vi "main-for-loop-V2.vi"() -> ()   [LabVIEW 2024]
uses:
  controls/thermocouple-input-cluster.ctl
  controls/analog-input-cluster.ctl
  controls/analog-output-cluster.ctl
  controls/digitial-input-cluster.ctl
  controls/digital-output-cluster.ctl
  controls/adam-module-select-tab.ctl
  controls/adam-5000-serial-settings.ctl
  controls/adam-5000-cmd-response.ctl
  controls/state-enum.ctl
  controls/adam-5000-all-chassis-data.ctl
  controls/adam-5000-all-module-datas.ctl
  controls/adam-5000-chassis-cmd-ack.ctl
  <vilib>/Instr/_visa.llb/VISA Configure Serial Port (Instr).vi
  <vilib>/Instr/_visa.llb/VISA Flush IO Buffer Mask.ctl
  controls/adam-5000-module-cmd-ack.ctl
panel:
  out "cmd-response:7":T1
  out "status-indicator:7":cluster{"Sampling":bool, "Ack":bool}
  in  "Slot 7: Module Type":T2(ring)=enum."empty"
  out "slot: 7":T3
  in  "7:Digital Outputs":T4
  out "7:Digital Inputs":T5
  in  "7:Analog Outputs":T6
  out "7:Analog Inputs":T7
  out "7:Thermocouple Inputs (degC)":T8
  out "cmd-response:6":T1
  out "status-indicator:6":cluster{"Sampling":bool, "Ack":bool}
  in  "Slot 6: Module Type":T2(ring)=enum."empty"
  out "slot: 6":T3
  in  "6:Digital Outputs":T4
  out "6:Digital Inputs":T5
  in  "6:Analog Outputs":T6
  out "6:Analog Inputs":T7
  out "6:Thermocouple Inputs (degC)":T8
  out "cmd-response:5":T1
  out "status-indicator:5":cluster{"Sampling":bool, "Ack":bool}
  in  "Slot 5: Module Type":T2(ring)=enum."Analog Output"
  out "slot: 5":T3
  in  "5:Digital Outputs":T4
  out "5:Digital Inputs":T5
  in  "5:Analog Outputs":T6
  out "5:Analog Inputs":T7
  out "5:Thermocouple Inputs (degC)":T8
  out "cmd-response:4":T1
  out "status-indicator:4":cluster{"Sampling":bool, "Ack":bool}
  in  "Slot 4: Module Type":T2(ring)=enum."Power Relay"
  out "slot: 4":T3
  in  "4:Digital Outputs":T4
  out "4:Digital Inputs":T5
  in  "4:Analog Outputs":T6
  out "4:Analog Inputs":T7
  out "4:Thermocouple Inputs (degC)":T8
  out "cmd-response:3":T1
  out "status-indicator:3":cluster{"Sampling":bool, "Ack":bool}
  in  "Slot 3: Module Type":T2(ring)=enum."Thermocouple"
  out "slot: 3":T3
  in  "3:Digital Outputs":T4
  out "3:Digital Inputs":T5
  in  "3:Analog Outputs":T6
  out "3:Analog Inputs":T7
  out "3:Thermocouple Inputs (degC)":T8
  out "cmd-response:2":T1
  out "status-indicator:2":cluster{"Sampling":bool, "Ack":bool}
  in  "Slot 2: Module Type":T2(ring)=enum."Analog Input"
  out "slot: 2":T3
  in  "2:Digital Outputs":T4
  out "2:Digital Inputs":T5
  in  "2:Analog Outputs":T6
  out "2:Analog Inputs":T7
  out "2:Thermocouple Inputs (degC)":T8
  out "cmd-response:1":T1
  out "status-indicator:1":cluster{"Sampling":bool, "Ack":bool}
  in  "Slot 1: Module Type":T2(ring)=enum."Thermocouple"
  out "slot: 1":T3
  in  "1:Digital Outputs":T4
  out "1:Digital Inputs":T5
  in  "1:Analog Outputs":T6
  out "1:Analog Inputs":T7
  out "1:Thermocouple Inputs (degC)":T8
  out "cmd-response:0":T1
  out "status-indicator:0":cluster{"Sampling":bool, "Ack":bool}
  in  "Slot 0: Module Type":T2(ring)=enum."Analog Input"
  out "slot: 0":T3
  in  "0:Digital Outputs":T4
  out "0:Digital Inputs":T5
  in  "0:Analog Outputs:":T6
  out "0:Analog Inputs":T7
  out "0:Thermocouple Inputs (degC)":T8
  out "Current Slot":i32
  in  "Chassis Settings":T9={"VISA resource name"="COM10", "baud rate (19200)"=19200, "Chassis ID"=1}
  in  "Debug Mode":bool
  out "Loop Time (mS)":u32
  out "Loop Counter":i32
  out "Write Success":bool
  out "error IO":errorcluster
  out "error":errorcluster
  in  "exit":bool
  # "ADAM 5000 Controller"
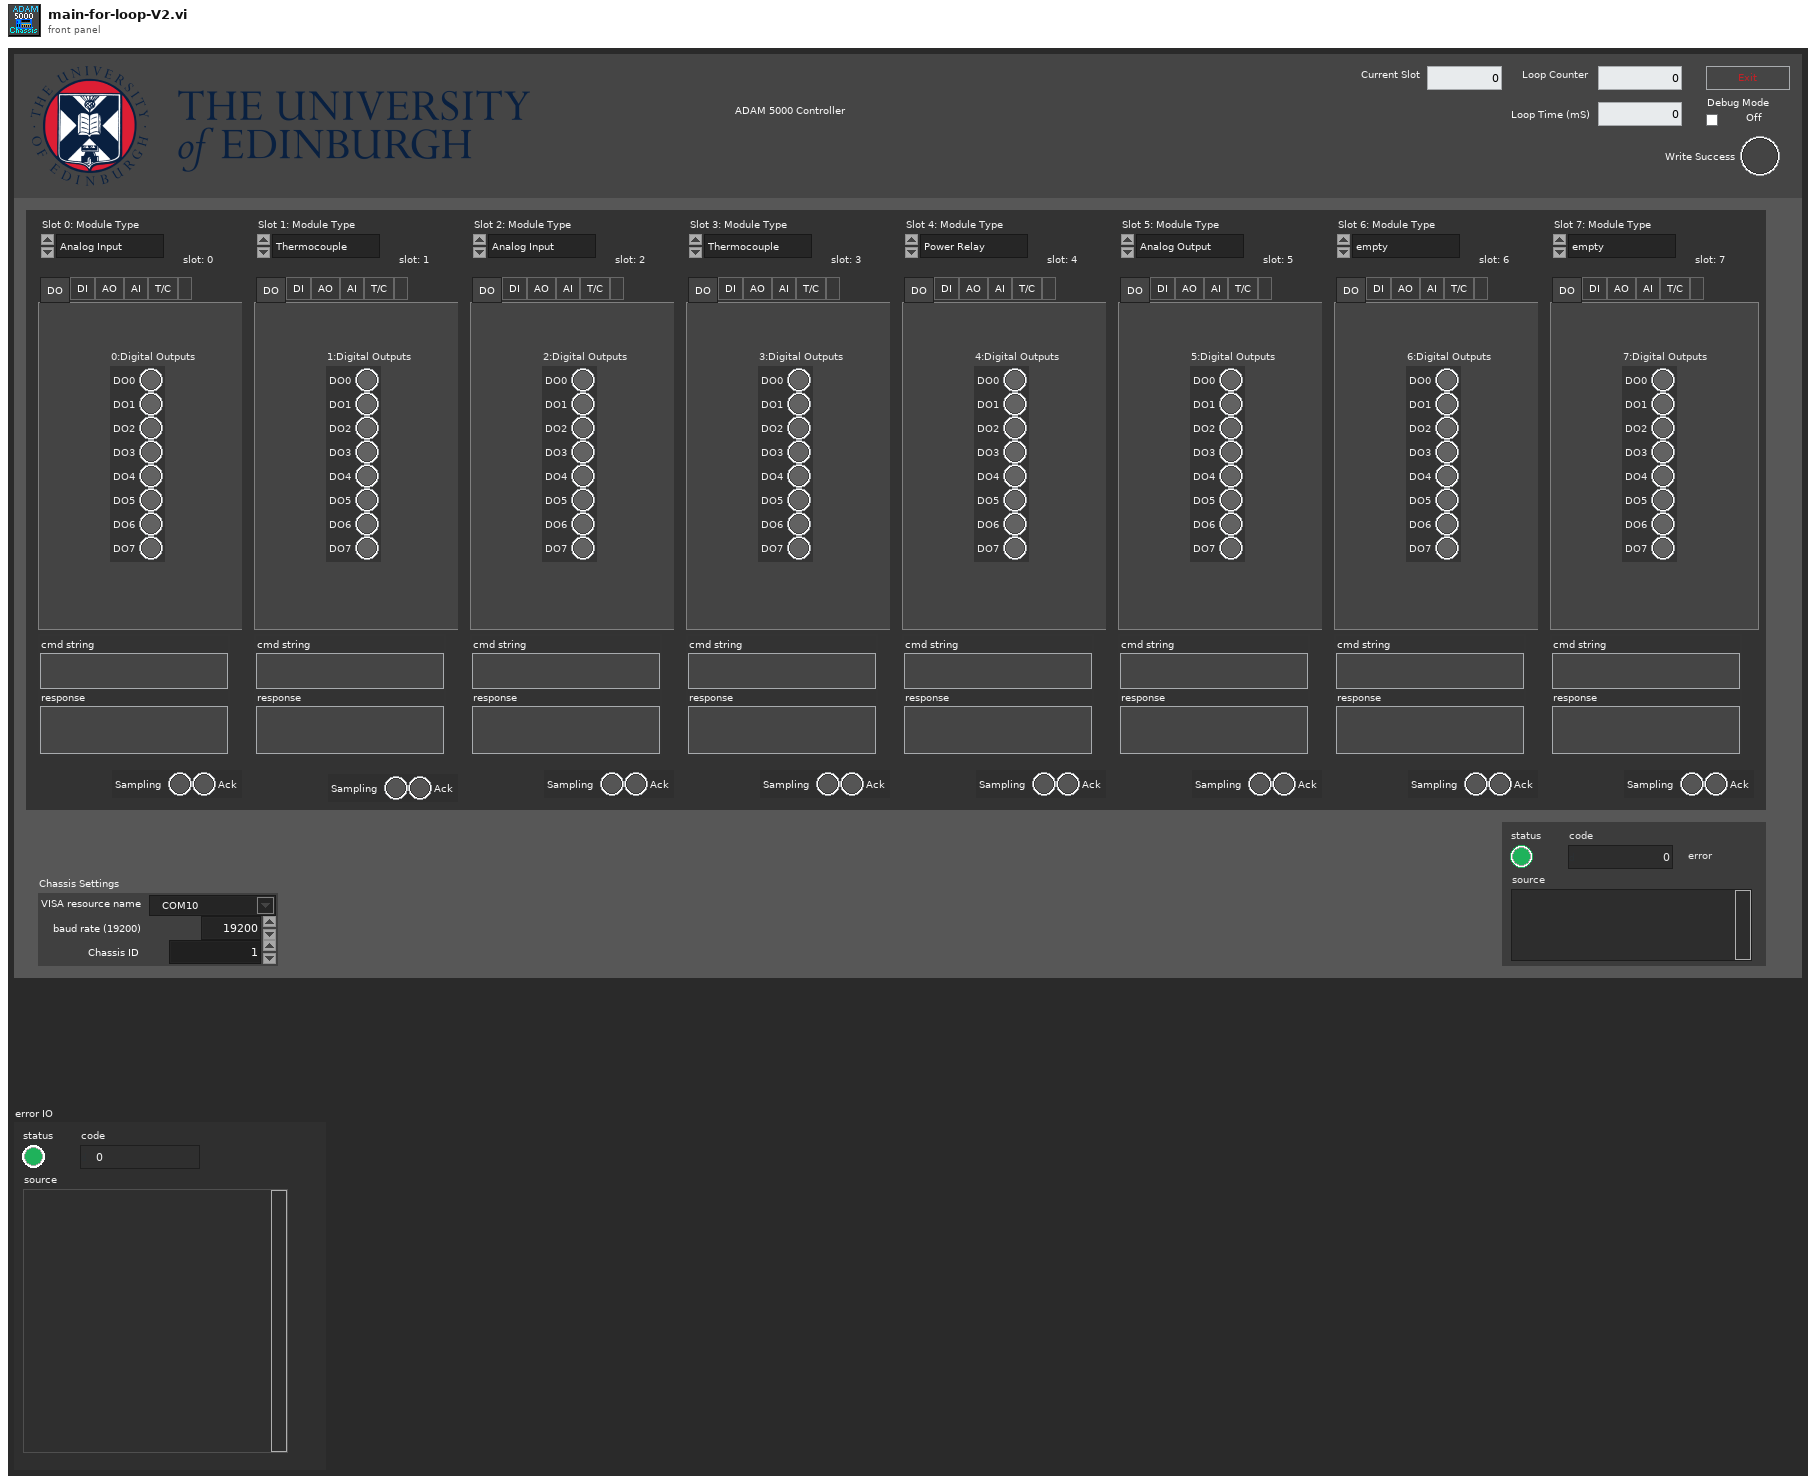
[diagram p1: front panel]
types:
  T1 = typedef "adam-5000-cmd-response.ctl" = cluster{"cmd string":string, "response":string}
  T2 = enum16{"Digital Output", "Digital Input", "Analog Output", "Analog Input", "Thermocouple", "Power Relay", "empty"}
  T3 = typedef "adam-module-select-tab.ctl" = enum32{"DO", "DI", "AO", "AI", "T/C", ""}
  T4 = typedef "digital-output-cluster.ctl" = cluster{"DO0":bool, "DO1":bool, "DO2":bool, "DO3":bool, "DO4":bool, "DO5":bool, "DO6":bool, "DO7":bool}
  T5 = typedef "digitial-input-cluster.ctl" = cluster{"DI0":bool, "DI1":bool, "DI2":bool, "DI3":bool, "DI4":bool, "DI5":bool, "DI6":bool, "DI7":bool}
  T6 = typedef "analog-output-cluster.ctl" = cluster{"AO0":dbl, "AO1":dbl, "AO2":dbl, "AO3":dbl}
  T7 = typedef "analog-input-cluster.ctl" = cluster{"AI0":dbl, "AI1":dbl, "AI2":dbl, "AI3":dbl, "AI4":dbl, "AI5":dbl, "AI6":dbl, "AI7":dbl}
  T8 = typedef "thermocouple-input-cluster.ctl" = cluster{"TC0":dbl, "TC1":dbl, "TC2":dbl, "TC3":dbl, "TC4":dbl, "TC5":dbl, "TC6":dbl}
  T9 = typedef "adam-5000-serial-settings.ctl" = cluster{"VISA resource name":refnum<visa-resource-name>, "baud rate (19200)":u32, "Chassis ID":u8}
  T10 = typedef "adam-5000-chassis-cmd-ack.ctl" = cluster{"cmd-response:0":T1, "cmd-response:1":T1, "cmd-response:2":T1, "cmd-response:3":T1, "cmd-response:4":T1, "cmd-response:5":T1, "cmd-response:6":T1, "cmd-response:7":T1}
  T11 = typedef "adam-5000-all-chassis-data.ctl" = cluster{"slot:0":T12, "slot:1":T12, "slot:2":T12, "slot:3":T12, "slot:4":T12, "slot:5":T12, "slot:6":T12, "slot:7":T12}
  T12 = typedef "adam-5000-all-module-datas.ctl" = cluster{"Digital Outputs":T4, "Digital Inputs":T5, "Analog Outputs":T6, "Analog Inputs":T7, "Thermocouple Inputs (degC)":T8}
  T13 = typedef "state-enum.ctl" = enum16{"init", "manual", "start", "run", "hold", "stop", ""}
  T14 = cluster{"0:Digital Outputs":T4, "1:Digital Outputs":T4, "2:Digital Outputs":T4, "3:Digital Outputs":T4, "4:Digital Outputs":T4, "5:Digital Outputs":T4, "6:Digital Outputs":T4, "7:Digital Outputs":T4}
  T15 = cluster{"Slot 0: Module Type":enum16{"Digital Output", "Digital Input", "Analog Output", "Analog Input", "Thermocouple", "Power Relay", "empty"}, "Slot 1: Module Type":enum16{"Digital Output", "Digital Input", "Analog Output", "Analog Input", "Thermocouple", "Power Relay", "empty"}, "Slot 2: Module Type":enum16{"Digital Output", "Digital Input", "Analog Output", "Analog Input", "Thermocouple", "Power Relay", "empty"}, "Slot 3: Module Type":enum16{"Digital Output", "Digital Input", "Analog Output", "Analog Input", "Thermocouple", "Power Relay", "empty"}, "Slot 4: Module Type":enum16{"Digital Output", "Digital Input", "Analog Output", "Analog Input", "Thermocouple", "Power Relay", "empty"}, "Slot 5: Module Type":enum16{"Digital Output", "Digital Input", "Analog Output", "Analog Input", "Thermocouple", "Power Relay", "empty"}, "Slot 6: Module Type":enum16{"Digital Output", "Digital Input", "Analog Output", "Analog Input", "Thermocouple", "Power Relay", "empty"}, "Slot 7: Module Type":enum16{"Digital Output", "Digital Input", "Analog Output", "Analog Input", "Thermocouple", "Power Relay", "empty"}}
  T16 = cluster{"status-indicator:0":refnum<vi>, "status-indicator:1":refnum<vi>, "status-indicator:2":refnum<vi>, "status-indicator:3":refnum<vi>, "status-indicator:4":refnum<vi>, "status-indicator:5":refnum<vi>, "status-indicator:6":refnum<vi>, "status-indicator:7":refnum<vi>}
  T17 = cluster{"0:Analog Outputs:":T6, "1:Analog Outputs":T6, "2:Analog Outputs":T6, "3:Analog Outputs":T6, "4:Analog Outputs":T6, "5:Analog Outputs":T6, "6:Analog Outputs":T6, "7:Analog Outputs":T6}
  T18 = enum16{"Digital Output", "Digital Input", "Analog Output", "Analog Input", "Thermocouple", "Power Relay", "empty"}[]
  T19 = cluster{"[0]":T3, "[1]":T3, "[2]":T3, "[3]":T3, "[4]":T3, "[5]":T3, "[6]":T3, "[7]":T3, "[8]":T3}
  T20 = cluster{"[0]":T1, "[1]":T1, "[2]":T1, "[3]":T1, "[4]":T1, "[5]":T1, "[6]":T1, "[7]":T1, "[8]":T1}
  T21 = cluster{"[0]":T12, "[1]":T12, "[2]":T12, "[3]":T12, "[4]":T12, "[5]":T12, "[6]":T12, "[7]":T12, "[8]":T12}
  T22 = typedef "adam-5000-module-cmd-ack.ctl" = cluster{"cmd out":string, "acknowledge char":string}
  T23 = cluster{"[0]":T22, "[1]":T22, "[2]":T22, "[3]":T22, "[4]":T22, "[5]":T22, "[6]":T22, "[7]":T22, "[8]":T22}
  T24 = typedef "VISA Flush IO Buffer Mask.ctl" = u16
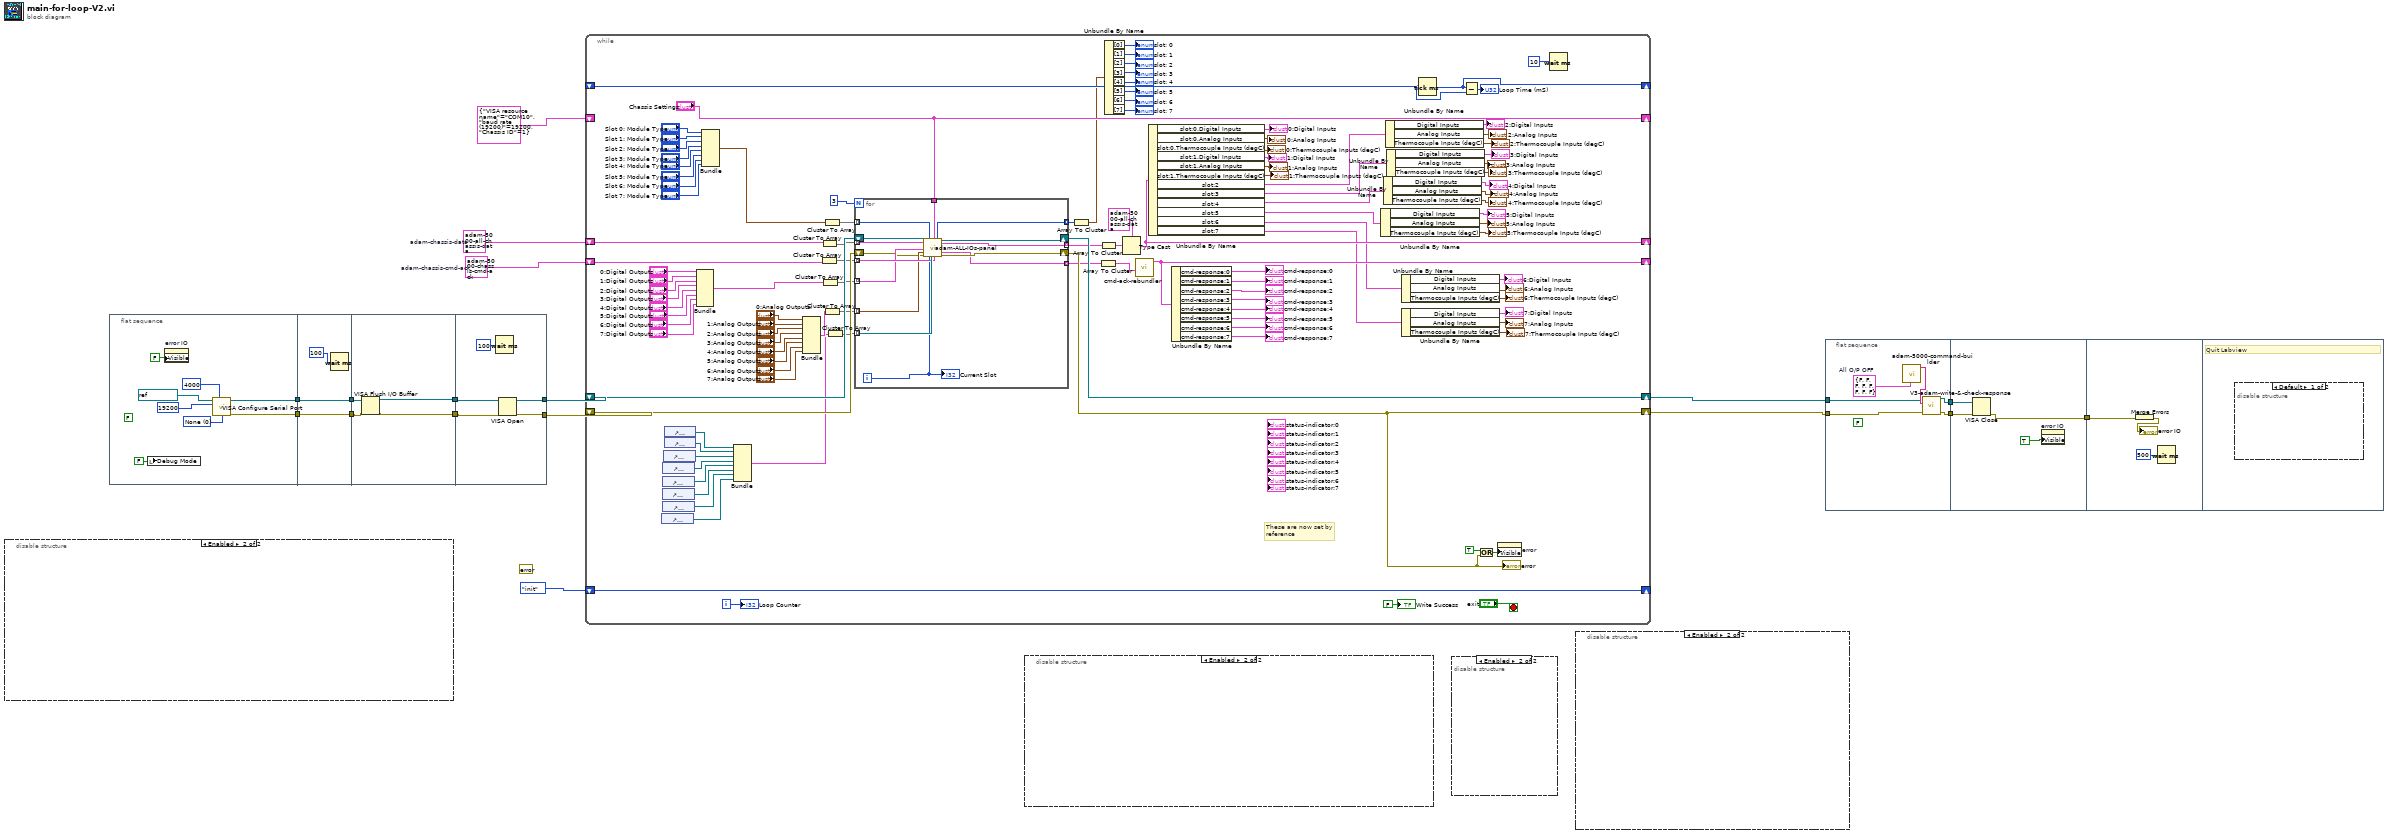
[diagram p0: block diagram]
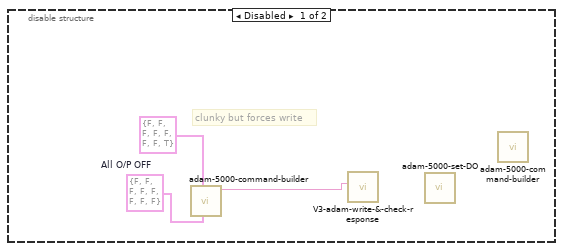
[diagram p2: hidden frame]
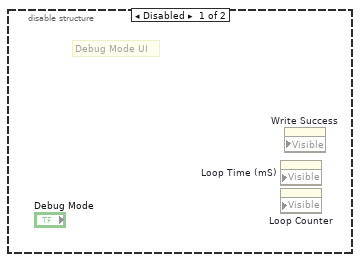
[diagram p3: hidden frame]
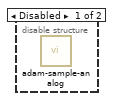
[diagram p4: hidden frame]
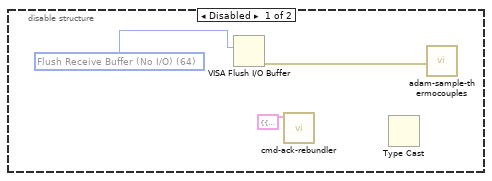
[diagram p5: hidden frame]
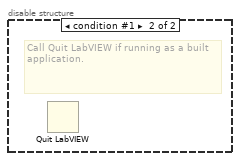
[diagram p6: hidden frame]
diagram:
  w1 = T10 {"cmd-response:0"={"cmd string"="", "response"=""}, "cmd-response:1"={"cmd string"="", "response"=""}, "cmd-response:2"={"cmd string"="", "response"=""}, "cmd-response:3"={"cmd string"="", "response"=""}, "cmd-response:4"={"cmd string"="", "response"=""}, "cmd-response:5"={"cmd string"="", "response"=""}, "cmd-response:6"={"cmd string"="", "response"=""}, "cmd-response:7"={"cmd string"="", "response"=""}}  # adam-chassis-cmd-ack
  w2 = T11 {"slot:0"={"Digital Outputs"={"DO0"=FALSE, "DO1"=FALSE, "DO2"=FALSE, "DO3"=FALSE, "DO4"=FALSE, "DO5"=FALSE, "DO6"=FALSE, "DO7"=FALSE}, "Digital Inputs"={"DI0"=FALSE, "DI1"=FALSE, "DI2"=FALSE, "DI3"=FALSE, "DI4"=FALSE, "DI5"=FALSE, "DI6"=FALSE, "DI7"=FALSE}, "Analog Outputs"={"AO0"=0.0, "AO1"=0.0, "AO2"=0.0, "AO3"=0.0}, "Analog Inputs"={"AI0"=0.0, "AI1"=0.0, "AI2"=0.0, "AI3"=0.0, "AI4"=0.0, "AI5"=0.0, "AI6"=0.0, "AI7"=0.0}, "Thermocouple Inputs (degC)"={"TC0"=0.0, "TC1"=0.0, "TC2"=0.0, "TC3"=0.0, "TC4"=0.0, "TC5"=0.0, "TC6"=0.0}}, "slot:1"={"Digital Outputs"={"DO0"=FALSE, "DO1"=FALSE, "DO2"=FALSE, "DO3"=FALSE, "DO4"=FALSE, "DO5"=FALSE, "DO6"=FALSE, "DO7"=FALSE}, "Digital Inputs"={"DI0"=FALSE, "DI1"=FALSE, "DI2"=FALSE, "DI3"=FALSE, "DI4"=FALSE, "DI5"=FALSE, "DI6"=FALSE, "DI7"=FALSE}, "Analog Outputs"={"AO0"=0.0, "AO1"=0.0, "AO2"=0.0, "AO3"=0.0}, "Analog Inputs"={"AI0"=0.0, "AI1"=0.0, "AI2"=0.0, "AI3"=0.0, "AI4"=0.0, "AI5"=0.0, "AI6"=0.0, "AI7"=0.0}, "Thermocouple Inputs (degC)"={"TC0"=0.0, "TC1"=0.0, "TC2"=0.0, "TC3"=0.0, "TC4"=0.0, "TC5"=0.0, "TC6"=0.0}}, "slot:2"={"Digital Outputs"={"DO0"=FALSE, "DO1"=FALSE, "DO2"=FALSE, "DO3"=FALSE, "DO4"=FALSE, "DO5"=FALSE, "DO6"=FALSE, "DO7"=FALSE}, "Digital Inputs"={"DI0"=FALSE, "DI1"=FALSE, "DI2"=FALSE, "DI3"=FALSE, "DI4"=FALSE, "DI5"=FALSE, "DI6"=FALSE, "DI7"=FALSE}, "Analog Outputs"={"AO0"=0.0, "AO1"=0.0, "AO2"=0.0, "AO3"=0.0}, "Analog Inputs"={"AI0"=0.0, "AI1"=0.0, "AI2"=0.0, "AI3"=0.0, "AI4"=0.0, "AI5"=0.0, "AI6"=0.0, "AI7"=0.0}, "Thermocouple Inputs (degC)"={"TC0"=0.0, "TC1"=0.0, "TC2"=0.0, "TC3"=0.0, "TC4"=0.0, "TC5"=0.0, "TC6"=0.0}}, "slot:3"={"Digital Outputs"={"DO0"=FALSE, "DO1"=FALSE, "DO2"=FALSE, "DO3"=FALSE, "DO4"=FALSE, "DO5"=FALSE, "DO6"=FALSE, "DO7"=FALSE}, "Digital Inputs"={"DI0"=FALSE, "DI1"=FALSE, "DI2"=FALSE, "DI3"=FALSE, "DI4"=FALSE, "DI5"=FALSE, "DI6"=FALSE, "DI7"=FALSE}, "Analog Outputs"={"AO0"=0.0, "AO1"=0.0, "AO2"=0.0, "AO3"=0.0}, "Analog Inputs"={"AI0"=0.0, "AI1"=0.0, "AI2"=0.0, "AI3"=0.0, "AI4"=0.0, "AI5"=0.0, "AI6"=0.0, "AI7"=0.0}, "Thermocouple Inputs (degC)"={"TC0"=0.0, "TC1"=0.0, "TC2"=0.0, "TC3"=0.0, "TC4"=0.0, "TC5"=0.0, "TC6"=0.0}}, "slot:4"={"Digital Outputs"={"DO0"=FALSE, "DO1"=FALSE, "DO2"=FALSE, "DO3"=FALSE, "DO4"=FALSE, "DO5"=FALSE, "DO6"=FALSE, "DO7"=FALSE}, "Digital Inputs"={"DI0"=FALSE, "DI1"=FALSE, "DI2"=FALSE, "DI3"=FALSE, "DI4"=FALSE, "DI5"=FALSE, "DI6"=FALSE, "DI7"=FALSE}, "Analog Outputs"={"AO0"=0.0, "AO1"=0.0, "AO2"=0.0, "AO3"=0.0}, "Analog Inputs"={"AI0"=0.0, "AI1"=0.0, "AI2"=0.0, "AI3"=0.0, "AI4"=0.0, "AI5"=0.0, "AI6"=0.0, "AI7"=0.0}, "Thermocouple Inputs (degC)"={"TC0"=0.0, "TC1"=0.0, "TC2"=0.0, "TC3"=0.0, "TC4"=0.0, "TC5"=0.0, "TC6"=0.0}}, "slot:5"={"Digital Outputs"={"DO0"=FALSE, "DO1"=FALSE, "DO2"=FALSE, "DO3"=FALSE, "DO4"=FALSE, "DO5"=FALSE, "DO6"=FALSE, "DO7"=FALSE}, "Digital Inputs"={"DI0"=FALSE, "DI1"=FALSE, "DI2"=FALSE, "DI3"=FALSE, "DI4"=FALSE, "DI5"=FALSE, "DI6"=FALSE, "DI7"=FALSE}, "Analog Outputs"={"AO0"=0.0, "AO1"=0.0, "AO2"=0.0, "AO3"=0.0}, "Analog Inputs"={"AI0"=0.0, "AI1"=0.0, "AI2"=0.0, "AI3"=0.0, "AI4"=0.0, "AI5"=0.0, "AI6"=0.0, "AI7"=0.0}, "Thermocouple Inputs (degC)"={"TC0"=0.0, "TC1"=0.0, "TC2"=0.0, "TC3"=0.0, "TC4"=0.0, "TC5"=0.0, "TC6"=0.0}}, "slot:6"={"Digital Outputs"={"DO0"=FALSE, "DO1"=FALSE, "DO2"=FALSE, "DO3"=FALSE, "DO4"=FALSE, "DO5"=FALSE, "DO6"=FALSE, "DO7"=FALSE}, "Digital Inputs"={"DI0"=FALSE, "DI1"=FALSE, "DI2"=FALSE, "DI3"=FALSE, "DI4"=FALSE, "DI5"=FALSE, "DI6"=FALSE, "DI7"=FALSE}, "Analog Outputs"={"AO0"=0.0, "AO1"=0.0, "AO2"=0.0, "AO3"=0.0}, "Analog Inputs"={"AI0"=0.0, "AI1"=0.0, "AI2"=0.0, "AI3"=0.0, "AI4"=0.0, "AI5"=0.0, "AI6"=0.0, "AI7"=0.0}, "Thermocouple Inputs (degC)"={"TC0"=0.0, "TC1"=0.0, "TC2"=0.0, "TC3"=0.0, "TC4"=0.0, "TC5"=0.0, "TC6"=0.0}}, "slot:7"={"Digital Outputs"={"DO0"=FALSE, "DO1"=FALSE, "DO2"=FALSE, "DO3"=FALSE, "DO4"=FALSE, "DO5"=FALSE, "DO6"=FALSE, "DO7"=FALSE}, "Digital Inputs"={"DI0"=FALSE, "DI1"=FALSE, "DI2"=FALSE, "DI3"=FALSE, "DI4"=FALSE, "DI5"=FALSE, "DI6"=FALSE, "DI7"=FALSE}, "Analog Outputs"={"AO0"=0.0, "AO1"=0.0, "AO2"=0.0, "AO3"=0.0}, "Analog Inputs"={"AI0"=0.0, "AI1"=0.0, "AI2"=0.0, "AI3"=0.0, "AI4"=0.0, "AI5"=0.0, "AI6"=0.0, "AI7"=0.0}, "Thermocouple Inputs (degC)"={"TC0"=0.0, "TC1"=0.0, "TC2"=0.0, "TC3"=0.0, "TC4"=0.0, "TC5"=0.0, "TC6"=0.0}}}  # adam-chassis-data
  (unwired) errorcluster {"status"=FALSE, "code"=0, "source"=""} ("error")
  n1 = disable-structure shown="Enabled" {
    frame Disabled {
      w20 = T4 {"DO0"=FALSE, "DO1"=FALSE, "DO2"=FALSE, "DO3"=FALSE, "DO4"=FALSE, "DO5"=FALSE, "DO6"=FALSE, "DO7"=FALSE}  # All O/P OFF
      # "clunky but forces write"
      n2 = call "adam-5000-command-builder.vi"("Output Control"=w20, "Current Output State"=T4 {"DO0"=FALSE, "DO1"=FALSE, "DO2"=FALSE, "DO3"=FALSE, "DO4"=FALSE, "DO5"=FALSE, "DO6"=FALSE, "DO7"=TRUE}) -> ("Command Out"=w19:string)  [unwired: 7 in, 2 out]
      n3 = call "V3-adam-write-&-check-response.vi"("write buffer"=w19) -> ("VISA resource name"=w18:refnum<visa-resource-name>)  [unwired: 5 in, 5 out]
      n4 = call "adam-5000-set-DO.vi"() -> ()  [unwired: 6 in, 6 out]
      n5 = call "adam-5000-command-builder.vi"() -> ()  [unwired: 9 in, 3 out]
    }
    frame Enabled {
    }
  }
  n6 = flat-sequence {
    tunnel: [w28] -> w11
    tunnel: [w27] -> w10
    tunnel: w11 -> [w32]
    tunnel: [w32] -> w9
    tunnel: w10 -> [w31]
    tunnel: [w31] -> w8
    tunnel: w9 -> [w36]
    tunnel: [w34] -> w7
    tunnel: w8 -> [w35]
    tunnel: [w33] -> w6
    tunnel: w7 -> [w40]
    tunnel: w6 -> [w39]
    tunnel: [w38] -> w5
    tunnel: [w37] -> w4
    frame #0 {
      w25 = u16 0 items=["None", "XON/XOFF", "RTS/CTS", "XON/XOFF & RTS/CTS", "DTR/DSR", "XON/XOFF & DTR/DSR"] ("flow control (0:none)")
      (unwired) FALSE ("V1")
      n7 = local write "Debug Mode"(FALSE ("Debug Mode")) -> ()
      n8 = property on="error IO" class="Clust (strict)"("Visible"=FALSE) -> ()  [unwired: 2 in, 2 out]
      n9 = call-poly "VISA Configure Serial Port"("VISA resource name"=refnum<visa-resource-name> "COM10", "timeout (10sec)"=u32 4000, "baud rate (9600)"=u32 19200, "flow control (0:none)"=w25) -> ("VISA resource name out"=w28:refnum<visa-resource-name>, "error out"=w27:errorcluster)  [unwired: 10 in]
    }
    frame #1 {
      n10 = Wait (ms)(milliseconds to wait=u32 100) -> ()  [unwired: 1 out]
    }
    frame #2 {
      n11 = VISA Flush I/O Buffer(VISA resource name=w36, error in (no error)=w35) -> (VISA resource name out=w34:refnum<visa-resource-name>, error out=w33:errorcluster)  [unwired: 1 in]
    }
    frame #3 {
      n12 = Wait (ms)(milliseconds to wait=u32 100) -> ()  [unwired: 1 out]
      n13 = VISA Open(error in (no error)=w39, VISA resource name=w40) -> (VISA resource name=w38:refnum<visa-resource-name>, error out=w37:errorcluster)  [unwired: 3 in]
    }
  }
  n14 = while {
    shift-right: [w148] -> _
    shift-left: state-enum."init" ("state-enum") -> [w148]
    shift-right: [w116] -> w16
    shift-left: w4 -> [w130]
    shift-right: [w151] -> _
    shift-left: _ -> [w153]
    shift-right: ["Chassis Settings"] -> _
    shift-left: T9 {"VISA resource name"="COM10", "baud rate (19200)"=19200, "Chassis ID"=1} ("Chassis Settings") -> [_]
    shift-right: [w129] -> w3
    shift-left: w5 -> [w131]
    shift-right: [w117] -> _
    shift-left: w2 -> [w128]
    shift-right: [w99] -> _
    shift-left: w1 -> [w126]
    i -> [w154]
    stop <- "exit" stop-if-true
    # "These are now set by\nreference"
    n15 = control-ref of="status-indicator:7"() -> (w42:refnum<vi>)
    n16 = control-ref of="status-indicator:4"() -> (w45:refnum<vi>)
    n17 = control-ref of="status-indicator:5"() -> (w44:refnum<vi>)
    n18 = control-ref of="status-indicator:3"() -> (w46:refnum<vi>)
    n19 = control-ref of="status-indicator:6"() -> (w43:refnum<vi>)
    n20 = control-ref of="status-indicator:2"() -> (w91:refnum<vi>)
    n21 = control-ref of="status-indicator:0"() -> (w112:refnum<vi>)
    n22 = control-ref of="status-indicator:1"() -> (w111:refnum<vi>)
    n23 = Bundle("0:Digital Outputs"="0:Digital Outputs", "1:Digital Outputs"="1:Digital Outputs", "2:Digital Outputs"="2:Digital Outputs", "3:Digital Outputs"="3:Digital Outputs", "4:Digital Outputs"="4:Digital Outputs", "5:Digital Outputs"="5:Digital Outputs", "6:Digital Outputs"="6:Digital Outputs", "7:Digital Outputs"="7:Digital Outputs") -> (w123:T14)  [unwired: 1 in]
    n24 = Bundle("Slot 0: Module Type"="Slot 0: Module Type", "Slot 1: Module Type"="Slot 1: Module Type", "Slot 2: Module Type"="Slot 2: Module Type", "Slot 3: Module Type"="Slot 3: Module Type", "Slot 4: Module Type"="Slot 4: Module Type", "Slot 5: Module Type"="Slot 5: Module Type", "Slot 6: Module Type"="Slot 6: Module Type", "Slot 7: Module Type"="Slot 7: Module Type") -> (w115:T15)  [unwired: 1 in]
    n25 = Bundle("status-indicator:0"=w112, "status-indicator:1"=w111, "status-indicator:2"=w91, "status-indicator:3"=w46, "status-indicator:4"=w45, "status-indicator:5"=w44, "status-indicator:6"=w43, "status-indicator:7"=w42) -> (w110:T16)  [unwired: 1 in]
    n26 = Bundle("0:Analog Outputs:"="0:Analog Outputs:", "1:Analog Outputs"="1:Analog Outputs", "2:Analog Outputs"="2:Analog Outputs", "3:Analog Outputs"="3:Analog Outputs", "4:Analog Outputs"="4:Analog Outputs", "5:Analog Outputs"="5:Analog Outputs", "6:Analog Outputs"="6:Analog Outputs", "7:Analog Outputs"="7:Analog Outputs") -> (w122:T17)  [unwired: 1 in]
    n27 = Cluster To Array(cluster=w126) -> (array=w125:T1[])
    n28 = Cluster To Array(cluster=w128) -> (array=w127:T12[])
    n29 = Cluster To Array(cluster=w123) -> (array=w124:T4[])
    n30 = Cluster To Array(cluster=w115) -> (array=w114:T18)
    n31 = Cluster To Array(cluster=w122) -> (array=w121:T6[])
    n32 = Cluster To Array(cluster=w110) -> (array=w109:refnum<vi>[])
    n33 = for {
      N: 3 -> [_]
      shift-right: [w160] -> w116
      shift-left: w130 -> [w161]
      shift-right: [w167] -> w129
      shift-left: w131 -> [w166]
      tunnel: w127 -> [w165] mode=indexing
      tunnel: w125 -> [w164] mode=indexing
      tunnel: w124 -> [w163] mode=indexing
      tunnel: w121 -> [w162] mode=indexing
      tunnel: "Chassis Settings" -> [w169]
      tunnel: w114 -> [w170] mode=indexing
      tunnel: w109 -> [w171] mode=indexing
      tunnel: [w168] -> w108 mode=indexing
      tunnel: [w159] -> w107 mode=indexing
      tunnel: [w158] -> w106 mode=indexing
      i -> [w157]
      n34 = call "adam-ALL-IOs-panel.vi"("VISA Refnum in"=w166, "ADAM-5000-data-current"=w165, "Digital Outputs"=w163, "Analog Outputs"=w162, "error in (no error)"=w161, "Module Type"=w170, "chassis-slot"=w157, "reference"=w171, "Chassis Settings"=w169, "cmd-response in"=w164) -> ("slot: x"=w168:T3, "VISA Refnum out"=w167:refnum<visa-resource-name>, "ADAM-5000-data-new"=w159:T12, "cmd-response out"=w158:T1, "error out"=w160:errorcluster)  [unwired: 5 in]
      "Current Slot" <- w157
    }
    "error" <- w116
    n35 = Array To Cluster(array=w108) -> (cluster=w113:T19)
    n36 = Array To Cluster(array=w106) -> (cluster=w98:T20)
    n37 = Array To Cluster(array=w107) -> (cluster=w119:T21)
    n38 = Unbundle By Name(w113) -> ("[0]"=→"slot: 0":T3, "[1]"=→"slot: 1":T3, "[2]"=→"slot: 2":T3, "[3]"=→"slot: 3":T3, "[4]"=→"slot: 4":T3, "[5]"=→"slot: 5":T3, "[6]"=→"slot: 6":T3, "[7]"=→"slot: 7":T3)
    n39 = Type Cast(type=T11 {"slot:0"={"Digital Outputs"={"DO0"=FALSE, "DO1"=FALSE, "DO2"=FALSE, "DO3"=FALSE, "DO4"=FALSE, "DO5"=FALSE, "DO6"=FALSE, "DO7"=FALSE}, "Digital Inputs"={"DI0"=FALSE, "DI1"=FALSE, "DI2"=FALSE, "DI3"=FALSE, "DI4"=FALSE, "DI5"=FALSE, "DI6"=FALSE, "DI7"=FALSE}, "Analog Outputs"={"AO0"=0.0, "AO1"=0.0, "AO2"=0.0, "AO3"=0.0}, "Analog Inputs"={"AI0"=0.0, "AI1"=0.0, "AI2"=0.0, "AI3"=0.0, "AI4"=0.0, "AI5"=0.0, "AI6"=0.0, "AI7"=0.0}, "Thermocouple Inputs (degC)"={"TC0"=0.0, "TC1"=0.0, "TC2"=0.0, "TC3"=0.0, "TC4"=0.0, "TC5"=0.0, "TC6"=0.0}}, "slot:1"={"Digital Outputs"={"DO0"=FALSE, "DO1"=FALSE, "DO2"=FALSE, "DO3"=FALSE, "DO4"=FALSE, "DO5"=FALSE, "DO6"=FALSE, "DO7"=FALSE}, "Digital Inputs"={"DI0"=FALSE, "DI1"=FALSE, "DI2"=FALSE, "DI3"=FALSE, "DI4"=FALSE, "DI5"=FALSE, "DI6"=FALSE, "DI7"=FALSE}, "Analog Outputs"={"AO0"=0.0, "AO1"=0.0, "AO2"=0.0, "AO3"=0.0}, "Analog Inputs"={"AI0"=0.0, "AI1"=0.0, "AI2"=0.0, "AI3"=0.0, "AI4"=0.0, "AI5"=0.0, "AI6"=0.0, "AI7"=0.0}, "Thermocouple Inputs (degC)"={"TC0"=0.0, "TC1"=0.0, "TC2"=0.0, "TC3"=0.0, "TC4"=0.0, "TC5"=0.0, "TC6"=0.0}}, "slot:2"={"Digital Outputs"={"DO0"=FALSE, "DO1"=FALSE, "DO2"=FALSE, "DO3"=FALSE, "DO4"=FALSE, "DO5"=FALSE, "DO6"=FALSE, "DO7"=FALSE}, "Digital Inputs"={"DI0"=FALSE, "DI1"=FALSE, "DI2"=FALSE, "DI3"=FALSE, "DI4"=FALSE, "DI5"=FALSE, "DI6"=FALSE, "DI7"=FALSE}, "Analog Outputs"={"AO0"=0.0, "AO1"=0.0, "AO2"=0.0, "AO3"=0.0}, "Analog Inputs"={"AI0"=0.0, "AI1"=0.0, "AI2"=0.0, "AI3"=0.0, "AI4"=0.0, "AI5"=0.0, "AI6"=0.0, "AI7"=0.0}, "Thermocouple Inputs (degC)"={"TC0"=0.0, "TC1"=0.0, "TC2"=0.0, "TC3"=0.0, "TC4"=0.0, "TC5"=0.0, "TC6"=0.0}}, "slot:3"={"Digital Outputs"={"DO0"=FALSE, "DO1"=FALSE, "DO2"=FALSE, "DO3"=FALSE, "DO4"=FALSE, "DO5"=FALSE, "DO6"=FALSE, "DO7"=FALSE}, "Digital Inputs"={"DI0"=FALSE, "DI1"=FALSE, "DI2"=FALSE, "DI3"=FALSE, "DI4"=FALSE, "DI5"=FALSE, "DI6"=FALSE, "DI7"=FALSE}, "Analog Outputs"={"AO0"=0.0, "AO1"=0.0, "AO2"=0.0, "AO3"=0.0}, "Analog Inputs"={"AI0"=0.0, "AI1"=0.0, "AI2"=0.0, "AI3"=0.0, "AI4"=0.0, "AI5"=0.0, "AI6"=0.0, "AI7"=0.0}, "Thermocouple Inputs (degC)"={"TC0"=0.0, "TC1"=0.0, "TC2"=0.0, "TC3"=0.0, "TC4"=0.0, "TC5"=0.0, "TC6"=0.0}}, "slot:4"={"Digital Outputs"={"DO0"=FALSE, "DO1"=FALSE, "DO2"=FALSE, "DO3"=FALSE, "DO4"=FALSE, "DO5"=FALSE, "DO6"=FALSE, "DO7"=FALSE}, "Digital Inputs"={"DI0"=FALSE, "DI1"=FALSE, "DI2"=FALSE, "DI3"=FALSE, "DI4"=FALSE, "DI5"=FALSE, "DI6"=FALSE, "DI7"=FALSE}, "Analog Outputs"={"AO0"=0.0, "AO1"=0.0, "AO2"=0.0, "AO3"=0.0}, "Analog Inputs"={"AI0"=0.0, "AI1"=0.0, "AI2"=0.0, "AI3"=0.0, "AI4"=0.0, "AI5"=0.0, "AI6"=0.0, "AI7"=0.0}, "Thermocouple Inputs (degC)"={"TC0"=0.0, "TC1"=0.0, "TC2"=0.0, "TC3"=0.0, "TC4"=0.0, "TC5"=0.0, "TC6"=0.0}}, "slot:5"={"Digital Outputs"={"DO0"=FALSE, "DO1"=FALSE, "DO2"=FALSE, "DO3"=FALSE, "DO4"=FALSE, "DO5"=FALSE, "DO6"=FALSE, "DO7"=FALSE}, "Digital Inputs"={"DI0"=FALSE, "DI1"=FALSE, "DI2"=FALSE, "DI3"=FALSE, "DI4"=FALSE, "DI5"=FALSE, "DI6"=FALSE, "DI7"=FALSE}, "Analog Outputs"={"AO0"=0.0, "AO1"=0.0, "AO2"=0.0, "AO3"=0.0}, "Analog Inputs"={"AI0"=0.0, "AI1"=0.0, "AI2"=0.0, "AI3"=0.0, "AI4"=0.0, "AI5"=0.0, "AI6"=0.0, "AI7"=0.0}, "Thermocouple Inputs (degC)"={"TC0"=0.0, "TC1"=0.0, "TC2"=0.0, "TC3"=0.0, "TC4"=0.0, "TC5"=0.0, "TC6"=0.0}}, "slot:6"={"Digital Outputs"={"DO0"=FALSE, "DO1"=FALSE, "DO2"=FALSE, "DO3"=FALSE, "DO4"=FALSE, "DO5"=FALSE, "DO6"=FALSE, "DO7"=FALSE}, "Digital Inputs"={"DI0"=FALSE, "DI1"=FALSE, "DI2"=FALSE, "DI3"=FALSE, "DI4"=FALSE, "DI5"=FALSE, "DI6"=FALSE, "DI7"=FALSE}, "Analog Outputs"={"AO0"=0.0, "AO1"=0.0, "AO2"=0.0, "AO3"=0.0}, "Analog Inputs"={"AI0"=0.0, "AI1"=0.0, "AI2"=0.0, "AI3"=0.0, "AI4"=0.0, "AI5"=0.0, "AI6"=0.0, "AI7"=0.0}, "Thermocouple Inputs (degC)"={"TC0"=0.0, "TC1"=0.0, "TC2"=0.0, "TC3"=0.0, "TC4"=0.0, "TC5"=0.0, "TC6"=0.0}}, "slot:7"={"Digital Outputs"={"DO0"=FALSE, "DO1"=FALSE, "DO2"=FALSE, "DO3"=FALSE, "DO4"=FALSE, "DO5"=FALSE, "DO6"=FALSE, "DO7"=FALSE}, "Digital Inputs"={"DI0"=FALSE, "DI1"=FALSE, "DI2"=FALSE, "DI3"=FALSE, "DI4"=FALSE, "DI5"=FALSE, "DI6"=FALSE, "DI7"=FALSE}, "Analog Outputs"={"AO0"=0.0, "AO1"=0.0, "AO2"=0.0, "AO3"=0.0}, "Analog Inputs"={"AI0"=0.0, "AI1"=0.0, "AI2"=0.0, "AI3"=0.0, "AI4"=0.0, "AI5"=0.0, "AI6"=0.0, "AI7"=0.0}, "Thermocouple Inputs (degC)"={"TC0"=0.0, "TC1"=0.0, "TC2"=0.0, "TC3"=0.0, "TC4"=0.0, "TC5"=0.0, "TC6"=0.0}}}, x=w119) -> (*(type *) &x=w117:T11)
    n40 = call "cmd-ack-rebundler.vi"("cmd-response-in"=w98) -> ("adam-chassis-cmd-response-out"=w99:T10)  [unwired: 10 in]
    n41 = Unbundle By Name(w117) -> ("slot:0.Digital Inputs"=→"0:Digital Inputs":T5, "slot:0.Analog Inputs"=→"0:Analog Inputs":T7, "slot:0.Thermocouple Inputs (degC)"=→"0:Thermocouple Inputs (degC)":T8, "slot:1.Digital Inputs"=→"1:Digital Inputs":T5, "slot:1.Analog Inputs"=→"1:Analog Inputs":T7, "slot:1.Thermocouple Inputs (degC)"=→"1:Thermocouple Inputs (degC)":T8, "slot:2"=w103:T12, "slot:3"=w94:T12, "slot:4"=w86:T12, "slot:5"=w58:T12, "slot:6"=w54:T12, "slot:7"=w53:T12)
    n42 = Unbundle By Name(w99) -> ("cmd-response:0"=→"cmd-response:0":T1, "cmd-response:1"=→"cmd-response:1":T1, "cmd-response:2"=→"cmd-response:2":T1, "cmd-response:3"=→"cmd-response:3":T1, "cmd-response:4"=→"cmd-response:4":T1, "cmd-response:5"=→"cmd-response:5":T1, "cmd-response:6"=→"cmd-response:6":T1, "cmd-response:7"=→"cmd-response:7":T1)
    n43 = Unbundle By Name(w58) -> ("Digital Inputs"=→"5:Digital Inputs":T5, "Analog Inputs"=→"5:Analog Inputs":T7, "Thermocouple Inputs (degC)"=→"5:Thermocouple Inputs (degC)":T8)
    n44 = Unbundle By Name(w86) -> ("Digital Inputs"=→"4:Digital Inputs":T5, "Analog Inputs"=→"4:Analog Inputs":T7, "Thermocouple Inputs (degC)"=→"4:Thermocouple Inputs (degC)":T8)
    n45 = Unbundle By Name(w103) -> ("Digital Inputs"=→"2:Digital Inputs":T5, "Analog Inputs"=→"2:Analog Inputs":T7, "Thermocouple Inputs (degC)"=→"2:Thermocouple Inputs (degC)":T8)
    n46 = Unbundle By Name(w94) -> ("Digital Inputs"=→"3:Digital Inputs":T5, "Analog Inputs"=→"3:Analog Inputs":T7, "Thermocouple Inputs (degC)"=→"3:Thermocouple Inputs (degC)":T8)
    n47 = Unbundle By Name(w54) -> ("Digital Inputs"=→"6:Digital Inputs":T5, "Analog Inputs"=→"6:Analog Inputs":T7, "Thermocouple Inputs (degC)"=→"6:Thermocouple Inputs (degC)":T8)
    n48 = Unbundle By Name(w53) -> ("Digital Inputs"=→"7:Digital Inputs":T5, "Analog Inputs"=→"7:Analog Inputs":T7, "Thermocouple Inputs (degC)"=→"7:Thermocouple Inputs (degC)":T8)
    n49 = Tick Count (ms)() -> (millisecond timer value=w151:u32)
    n50 = Subtract(x=w151, y=w153) -> (x-y=→"Loop Time (mS)":u32)
    n51 = Or(x=TRUE ("Debug Mode"), y=w116) -> (x .or. y?=w150:bool)
    n52 = property on="error" class="Clust (strict)"("Visible"=w150) -> ()  [unwired: 2 in, 2 out]
    n53 = Wait (ms)(milliseconds to wait=u32 10) -> ()  [unwired: 1 out]
    "Write Success" <- FALSE ("Write Success")
    "Loop Counter" <- w154
  }
  n54 = disable-structure shown="Enabled" {
    frame Disabled {
      w177 = T24 64 items=["Flush Receive Buffer"=16, "Write Transmit Buffer to Device"=32, "Flush Receive Buffer (No I/O)"=64, "Flush Transmit Buffer"=128] ("Mask")
      n55 = VISA Flush I/O Buffer(mask (16)=w177) -> (error out=w176:errorcluster)  [unwired: 2 in, 1 out]
      n56 = call "cmd-ack-rebundler.vi"("adam-chassis-cmd-response-in"=T23 {"[0]"={"cmd out"="", "acknowledge char"=""}, "[1]"={"cmd out"="", "acknowledge char"=""}, "[2]"={"cmd out"="", "acknowledge char"=""}, "[3]"={"cmd out"="", "acknowledge char"=""}, "[4]"={"cmd out"="", "acknowledge char"=""}, "[5]"={"cmd out"="", "acknowledge char"=""}, "[6]"={"cmd out"="", "acknowledge char"=""}, "[7]"={"cmd out"="", "acknowledge char"=""}, "[8]"={"cmd out"="", "acknowledge char"=""}} ("cmd-ack-in")) -> ()  [unwired: 10 in, 1 out]
      n57 = Type Cast() -> ()  [unwired: 2 in, 1 out]
      n58 = call "adam-sample-thermocouples.vi"("error in (no error)"=w176) -> ("status"=w174:string, "read buffer"=w173:string, "acknowledge char"=w175:string)  [unwired: 5 in, 3 out]
    }
    frame Enabled {
    }
  }
  n59 = disable-structure shown="Enabled" {
    frame Disabled {
      n60 = call "adam-sample-analog.vi"() -> ()  [unwired: 6 in, 6 out]
    }
    frame Enabled {
    }
  }
  n61 = disable-structure shown="Enabled" {
    frame Disabled {
      # "Debug Mode UI"
      n62 = property on="Loop Time (mS)" class="DigNum (strict)" props=["Visible"]() -> ()  [unwired: 3 in, 2 out]
      n63 = property on="Loop Counter" class="DigNum (strict)" props=["Visible"]() -> ()  [unwired: 3 in, 2 out]
      n64 = property on="Write Success" class="Bool (strict)" props=["Visible"]() -> ()  [unwired: 3 in, 2 out]
    }
    frame Enabled {
    }
  }
  n65 = flat-sequence {
    tunnel: w16 -> [w183]
    tunnel: [w182] -> w14
    tunnel: [w181] -> w13
    tunnel: w3 -> [w179]
    tunnel: [w185] -> w15
    tunnel: w14 -> [w186]
    tunnel: w13 -> [w187]
    tunnel: w15 -> [w189]
    frame #0 {
      (unwired) FALSE ("V1")
      w180 = T4 {"DO0"=FALSE, "DO1"=FALSE, "DO2"=FALSE, "DO3"=FALSE, "DO4"=FALSE, "DO5"=FALSE, "DO6"=FALSE, "DO7"=FALSE}  # All O/P OFF
      n66 = call "adam-5000-command-builder.vi"("Output Control"=w180) -> ("Command Out"=w184:string)  [unwired: 8 in, 2 out]
      n67 = call "V3-adam-write-&-check-response.vi"("error in (no error)"=w183, "write buffer"=w184, "VISA resource name"=w179) -> ("error out"=w181:errorcluster, "VISA resource name out"=w182:refnum<visa-resource-name>)  [unwired: 4 in, 3 out]
    }
    frame #1 {
      n68 = VISA Close(VISA resource name=w186, error in (no error)=w187) -> (error out=w185:errorcluster)
      n69 = property on="error IO" class="Clust (strict)"("Visible"=TRUE) -> ()  [unwired: 2 in, 2 out]
    }
    frame #2 {
      n70 = Merge Errors(w189) -> (→"error IO":errorcluster)
      n71 = Wait (ms)(milliseconds to wait=u32 500) -> ()  [unwired: 1 out]
    }
    frame #3 {
      # "Quit Labview"
      n72 = disable-structure "Conditional Disable Structure" shown="Default" {
        frame condition #0 (active) {
        }
        frame condition #1 {
          # "Call Quit LabVIEW if running as a built application."
          n73 = Quit LabVIEW() -> ()  [unwired: 1 in]
        }
      }
    }
  }
